vi "SportTrack.vi"() -> ()   [LabVIEW 2023]
uses:
  Global_var.vi
  <vilib>/Utility/NIReport.llb/Report Type.ctl
  <vilib>/Utility/NIReport.llb/NI_ReportGenerationCore.lvlib
  <vilib>/Utility/NIReport.llb/NI_report.lvclass
  <vilib>/addons/_office/NI_ReportGenerationToolkit.lvlib
  <vilib>/addons/_office/word.llb/Word Find & Replace (str).vi
  <vilib>/Utility/NIReport.llb/Word/NI_Word.lvclass
  <vilib>/addons/_office/word.llb/Word Find & Replace (num).vi
  <vilib>/Instr/_visa.llb/VISA Configure Serial Port (Instr).vi
panel:
  out "Buffer vidé\nNe pas lancer tant que ce n'est pas vert constant !":bool
  out "Timer Value":dbl
  out "Execution Time":u32
  in  "stop":bool
  out "String reçu":string
  out "String decouper":string
  in  "OK Button":bool
  in  "time s":dbl min=0.0 max=10.0 step=1.0
  out "?":bool
  in  "acceleration input x (volt)":dbl=1.29 min=0.1 max=2.8 step=0.1
  in  "acceleration input y (volt)":dbl=1.29 min=0.1 max=2.8 step=0.1
  in  "acceleration input z (volt)":dbl=1.35 min=0.1 max=2.8 step=0.1
  out "ACC X":bool
  out "ACC Y":bool
  out "ACC Z":bool
  in  "VISA resource name":refnum<visa-resource-name>="COM7"
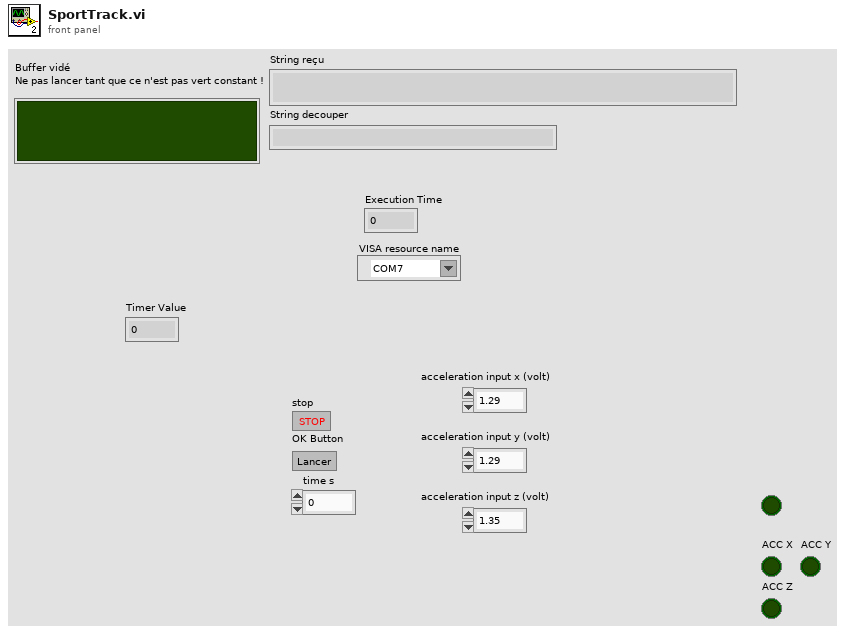
[diagram p1: front panel]
types:
  T1 = enum16{"maximized", "minimized", "normal", "no change"}
  T2 = typedef "NI_ReportGenerationCore.lvlib/Report Type.ctl" = enum16{"HTML", "Word", "Excel"}
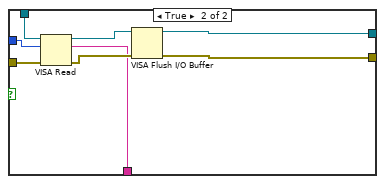
[diagram p2: hidden frame]
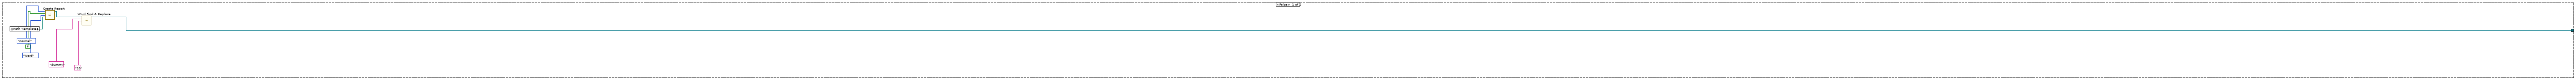
[diagram p4: hidden frame]
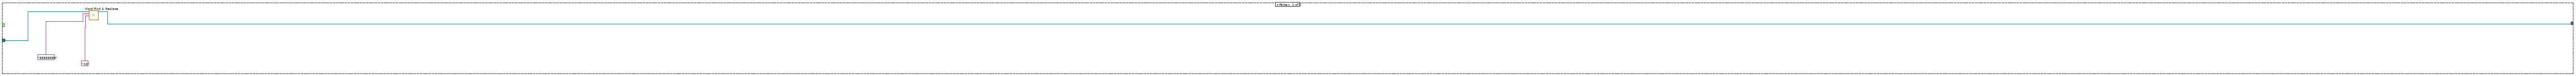
[diagram p5: hidden frame]
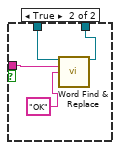
[diagram p6: hidden frame]
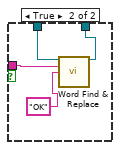
[diagram p7: hidden frame]
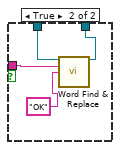
[diagram p8: hidden frame]
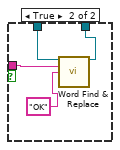
[diagram p9: hidden frame]
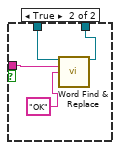
[diagram p10: hidden frame]
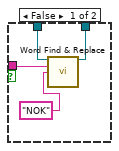
[diagram p11: hidden frame]
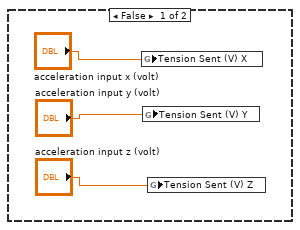
[diagram p12: hidden frame]
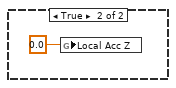
[diagram p13: hidden frame]
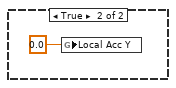
[diagram p14: hidden frame]
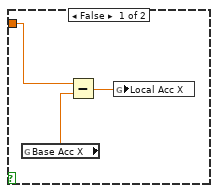
[diagram p15: hidden frame]
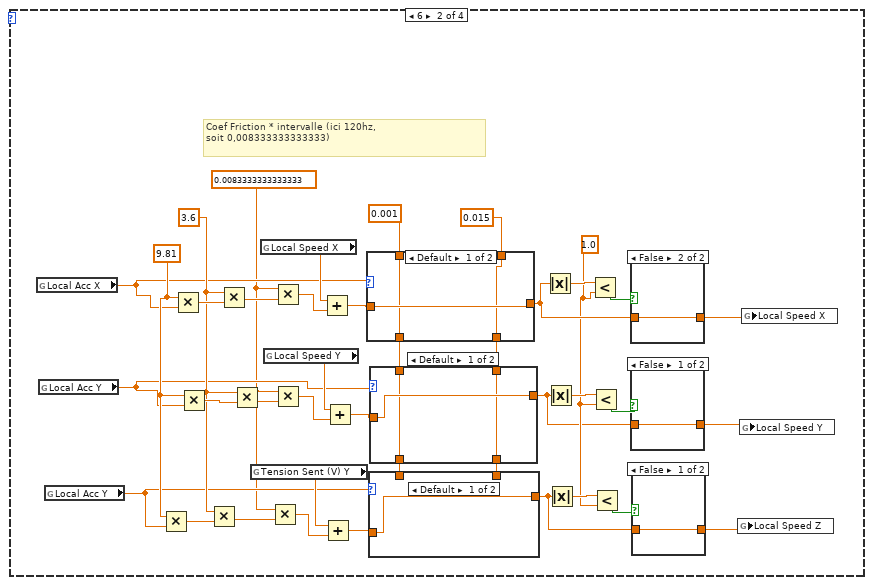
[diagram p17: hidden frame]
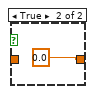
[diagram p18: hidden frame]
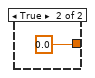
[diagram p19: hidden frame]
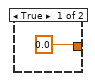
[diagram p20: hidden frame]
diagram:
  w25 = 240.0
  w9 = 0.0
  # "INITIALISATION DES VARIABLES"
  # "0G Voltage Z"
  # "0G Voltage Y"
  # "0G Voltage X"
  n1 = global write "Global_var.vi" "Speed Instant X"(w9) -> ()
  n2 = global write "Global_var.vi" "Speed Instant Y"(w9) -> ()
  n3 = global write "Global_var.vi" "Speed Instant Z"(w9) -> ()
  n4 = global write "Global_var.vi" "Local Speed X"(w9) -> ()
  n5 = global write "Global_var.vi" "Local Speed Y"(w9) -> ()
  n6 = global write "Global_var.vi" "Local Speed Z"(w9) -> ()
  n7 = global write "Global_var.vi" "Local Acc X"(w9) -> ()
  n8 = global write "Global_var.vi" "Local Acc Z"(w9) -> ()
  n9 = global write "Global_var.vi" "Local Acc Y"(w9) -> ()
  n10 = global write "Global_var.vi" "Mesure"(0.0 ("Base Acc Z")) -> ()
  n11 = global write "Global_var.vi" "Acc X"(w9) -> ()
  n12 = global write "Global_var.vi" "Acc Y"(w9) -> ()
  n13 = global write "Global_var.vi" "Acc Z"(w9) -> ()
  n14 = call-poly "VISA Configure Serial Port"("VISA resource name"="VISA resource name", "baud rate (9600)"=115200) -> ("VISA resource name out"=w6:refnum<visa-resource-name>, "error out"=w5:errorcluster)  [unwired: 12 in]
  n15 = global read "Global_var.vi" "Base Tension (V) X"() -> (w10:dbl)
  n16 = global read "Global_var.vi" "Base Tension (V) Z"() -> (w12:dbl)
  n17 = global read "Global_var.vi" "Base Tension (V) Y"() -> (w11:dbl)
  n18 = VISA Clear(VISA resource name=w6, error in (no error)=w5) -> (VISA resource name out=w8:refnum<visa-resource-name>, error out=w7:errorcluster)
  n19 = VISA Open(error in (no error)=w7, VISA resource name=w8) -> (VISA resource name=w3:refnum<visa-resource-name>, error out=w4:errorcluster)  [unwired: 3 in]
  n20 = Current VI's Path() -> (path=w18:path)
  n21 = global write "Global_var.vi" "Base Tension (V) Z"(1.35) -> ()
  n22 = global write "Global_var.vi" "Base Tension (V) Y"(1.29) -> ()
  n23 = global write "Global_var.vi" "Base Tension (V) X"(1.29) -> ()
  n24 = Subtract(x=w11, y=1.29) -> (x-y=w26:dbl)
  n25 = Subtract(x=w10, y=1.29) -> (x-y=w30:dbl)
  n26 = Subtract(x=w12, y=1.35) -> (x-y=w27:dbl)
  n27 = Strip Path(path=w18) -> (stripped path=w21:path)  [unwired: 1 out]
  n28 = Divide(x=w26, y=w25) -> (x/y=w23:dbl)
  n29 = Divide(x=w30, y=w25) -> (x/y=w24:dbl)
  n30 = Divide(x=w27, y=w25) -> (x/y=w22:dbl)
  n31 = VISA Set I/O Buffer Size(VISA resource name=w3, mask (16)=16, size (4096)=5, error in (no error)=w4) -> (VISA resource name out=w2:refnum<visa-resource-name>, error out=w1:errorcluster)
  n32 = global write "Global_var.vi" "Base Acc X"(w24) -> ()
  n33 = global write "Global_var.vi" "Base Acc Y"(w23) -> ()
  n34 = global write "Global_var.vi" "Base Acc Z"(w22) -> ()
  n35 = Build Path(base path=w21, name or relative path=path "Mesures_LabVIEW.docx") -> (appended path=w16:path)
  n36 = Build Path(base path=w21, name or relative path=path "Rapport/Rapport.docx") -> (appended path=w17:path)
  n37 = global write "Global_var.vi" "Path Save"(w17) -> ()
  n38 = global write "Global_var.vi" "Path Template"(w16) -> ()
  n39 = while {
    shift-right: [w46] -> w39
    shift-left: w2 -> [w45]
    shift-right: [w47] -> w38
    shift-left: w1 -> [w44]
    tunnel: [w48] -> w14
    stop <- "stop" stop-if-true
    n40 = flat-sequence {
      tunnel: [w54] -> w51
      tunnel: [w99] -> w48
      tunnel: [w76] -> w46
      tunnel: [w75] -> w47
      tunnel: w43 -> [w60]
      tunnel: w42 -> [w61]
      tunnel: w41 -> [w59]
      tunnel: [w633] -> w52
      frame #0 {
        # "Starting Ticks"
        n41 = Tick Count (ms)() -> (millisecond timer value=w54:u32)
      }
      frame #1 {
        w150 = 0.05
        w162 = 0.05
        w174 = 0.05
        w182 = 0.24
        # "Acc z"
        # "mode"
        # "Acc y"
        # "Acc x"
        # "Speed z"
        # "Speed y"
        # "Speed x"
        # "valeurs en variable"
        # "CALCUL VITESSE"
        # "CALCUL ACCELERATION"
        n42 = Greater?(x=w60, y=100) -> (0:w64:bool)
        n43 = global read "Global_var.vi" "Tension Sent (V) Z"() -> (w86:dbl)
        n44 = global read "Global_var.vi" "Tension Sent (V) Y"() -> (w85:dbl)
        n45 = global read "Global_var.vi" "Tension Sent (V) X"() -> (w84:dbl)
        n46 = local read "String reçu"() -> (w58:string)
        n47 = Subtract(x=w85, y=1.29) -> (x-y=w183:dbl)
        n48 = Subtract(x=w86, y=1.35) -> (x-y=w184:dbl)
        n49 = Subtract(x=w84, y=1.29) -> (x-y=w187:dbl)
        n50 = global read "Global_var.vi" "Base Acc X"() -> (w170:dbl)
        n51 = Divide(x=w187, y=w182) -> (x/y=w83:dbl)
        n52 = Divide(x=w183, y=w182) -> (x/y=w81:dbl)
        n53 = Divide(x=w184, y=w182) -> (x/y=w79:dbl)
        n54 = global read "Global_var.vi" "Base Acc Y"() -> (w158:dbl)
        n55 = global read "Global_var.vi" "Base Acc Z"() -> (w146:dbl)
        n56 = call <vilib>:"Trim Whitespace.vi"("string"=w58) -> ("trimmed string"=w144:string)  [unwired: 1 in]
        n57 = Absolute Value(x=w170) -> (abs(x)=w179:dbl)
        n58 = Absolute Value(x=w170) -> (abs(x)=w181:dbl)
        n59 = Absolute Value(x=w158) -> (abs(x)=w167:dbl)
        n60 = Absolute Value(x=w158) -> (abs(x)=w169:dbl)
        n61 = Match Pattern(string=w144, regular expression="x:") -> (before substring=w67:string, after substring=w141:string)  [unwired: 1 in, 2 out]
        n62 = Equal?(x="SI: ", y=w67) -> (x = y?=w62:bool)
        n63 = And(x=w64, y=w62) -> (x .and. y?=w57:bool)
        n64 = Not(x=w57) -> (.not. x?=→"Buffer vidé\nNe pas lancer tant que ce n'est pas vert constant !":bool)
        n65 = case shown="False" w57 {
          tunnel: [w191 w202] -> w66
          tunnel: [w190 w201] -> w65
          tunnel: w61 -> [w193 w200]
          tunnel: w60 -> [w192 w199]
          tunnel: w59 -> [w194 w198]
          tunnel: [w189 w195] -> w55
          frame False {
            n66 = VISA Read(VISA resource name=w194, byte count=w192, error in (no error)=w193) -> (VISA resource name out=w190:refnum<visa-resource-name>, read buffer=w189:string, error out=w191:errorcluster)  [unwired: 1 out]
          }
          frame True {
            n67 = VISA Read(VISA resource name=w198, byte count=w199, error in (no error)=w200) -> (VISA resource name out=w196:refnum<visa-resource-name>, read buffer=w195:string, error out=w197:errorcluster)  [unwired: 1 out]
            n68 = VISA Flush I/O Buffer(VISA resource name=w196, error in (no error)=w197) -> (VISA resource name out=w201:refnum<visa-resource-name>, error out=w202:errorcluster)  [unwired: 1 in]
          }
        }
        "String reçu" <- w55
        n69 = Multiply(x=1.05, y=w179) -> (x*y=w177:dbl)
        n70 = Multiply(x=0.95, y=w181) -> (x*y=w176:dbl)
        n71 = Absolute Value(x=w146) -> (abs(x)=w155:dbl)
        n72 = Absolute Value(x=w146) -> (abs(x)=w157:dbl)
        n73 = Multiply(x=1.05, y=w167) -> (x*y=w165:dbl)
        n74 = Multiply(x=0.95, y=w169) -> (x*y=w164:dbl)
        n75 = Multiply(x=1.05, y=w155) -> (x*y=w153:dbl)
        n76 = Subtract(x=w174, y=w176) -> (x-y=w175:dbl)
        n77 = Add(x=w174, y=w177) -> (x+y=w171:dbl)
        n78 = Multiply(x=0.95, y=w157) -> (x*y=w152:dbl)
        n79 = Absolute Value(x=w83) -> (abs(x)=w82:dbl)
        n80 = Subtract(x=w162, y=w164) -> (x-y=w163:dbl)
        n81 = Add(x=w162, y=w165) -> (x+y=w159:dbl)
        n82 = Subtract(x=w150, y=w152) -> (x-y=w151:dbl)
        n83 = Add(x=w150, y=w153) -> (x+y=w147:dbl)
        n84 = Absolute Value(x=w81) -> (abs(x)=w80:dbl)
        n85 = call <vilib>:"Trim Whitespace.vi"("string"=w141) -> ("trimmed string"=w140:string)  [unwired: 1 in]
        n86 = Match Pattern(string=w140, regular expression="y:") -> (before substring=w97:string, after substring=w137:string)  [unwired: 1 in, 2 out]
        n87 = call <vilib>:"Trim Whitespace.vi"("string"=w137) -> ("trimmed string"=w138:string)  [unwired: 1 in]
        n88 = Match Pattern(string=w138, regular expression="z:") -> (before substring=w96:string, after substring=w132:string)  [unwired: 1 in, 2 out]
        n89 = call <vilib>:"Trim Whitespace.vi"("string"=w132) -> ("trimmed string"=w135:string)  [unwired: 1 in]
        n90 = Match Pattern(string=w135, regular expression="A: x:") -> (before substring=w95:string, after substring=w131:string)  [unwired: 1 in, 2 out]
        n91 = call <vilib>:"Trim Whitespace.vi"("string"=w131) -> ("trimmed string"=w133:string)  [unwired: 1 in]
        n92 = Match Pattern(string=w133, regular expression="y:") -> (before substring=w98:string, after substring=w129:string)  [unwired: 1 in, 2 out]
        n93 = call <vilib>:"Trim Whitespace.vi"("string"=w129) -> ("trimmed string"=w122:string)  [unwired: 1 in]
        n94 = Match Pattern(string=w122, regular expression="z:") -> (before substring=w69:string, after substring=w121:string)  [unwired: 1 in, 2 out]
        n95 = call <vilib>:"Trim Whitespace.vi"("string"=w121) -> ("trimmed string"=w120:string)  [unwired: 1 in]
        n96 = Match Pattern(string=w120, regular expression="M:") -> (before substring=w70:string, after substring=w119:string)  [unwired: 1 in, 2 out]
        n97 = Absolute Value(x=w79) -> (abs(x)=w78:dbl)
        n98 = Greater Or Equal?(x=w82, y=w175) -> (x >= y?=w172:bool)
        n99 = Less Or Equal?(x=w82, y=w171) -> (x <= y?=w173:bool)
        n100 = Greater Or Equal?(x=w80, y=w163) -> (x >= y?=w160:bool)
        n101 = Less Or Equal?(x=w80, y=w159) -> (x <= y?=w161:bool)
        n102 = And(x=w173, y=w172) -> (x .and. y?=w104:bool)
        "ACC X" <- w104
        n103 = Greater Or Equal?(x=w78, y=w151) -> (x >= y?=w148:bool)
        n104 = Less Or Equal?(x=w78, y=w147) -> (x <= y?=w149:bool)
        n105 = And(x=w161, y=w160) -> (x .and. y?=w105:bool)
        "ACC Y" <- w105
        n106 = And(x=w149, y=w148) -> (x .and. y?=w106:bool)
        "ACC Z" <- w106
        n107 = Concatenate Strings(w97, w96, w95, w98, w69, w70, w119) -> (→"String decouper":string)
        n108 = case shown="True" w104 {
          tunnel: w83 -> [w494 _]
          frame False {
            n109 = global read "Global_var.vi" "Base Acc X"() -> (w493:dbl)
            n110 = Subtract(x=w494, y=w493) -> (x-y=w495:dbl)
            n111 = global write "Global_var.vi" "Local Acc X"(w495) -> ()
          }
          frame True {
            n112 = global write "Global_var.vi" "Local Acc X"(0.0) -> ()
          }
        }
        n113 = case shown="False" w106 {
          tunnel: w79 -> [w486 _]
          frame False {
            n114 = global read "Global_var.vi" "Base Acc Z"() -> (w485:dbl)
            n115 = Subtract(x=w486, y=w485) -> (x-y=w487:dbl)
            n116 = global write "Global_var.vi" "Local Acc Z"(w487) -> ()
          }
          frame True {
            n117 = global write "Global_var.vi" "Local Acc Z"(0.0) -> ()
          }
        }
        n118 = case shown="False" w105 {
          tunnel: w81 -> [w490 _]
          frame False {
            n119 = global read "Global_var.vi" "Base Acc Y"() -> (w489:dbl)
            n120 = Subtract(x=w490, y=w489) -> (x-y=w491:dbl)
            n121 = global write "Global_var.vi" "Local Acc Y"(w491) -> ()
          }
          frame True {
            n122 = global write "Global_var.vi" "Local Acc Y"(0.0) -> ()
          }
        }
        n123 = String Subset(string=w119) -> (substring=w127:string)  [unwired: 2 in]
        n124 = Fract/Exp String To Number(use system decimal point (T)=FALSE, string=w98) -> (number=w113:dbl)  [unwired: 2 in, 1 out]
        n125 = Fract/Exp String To Number(use system decimal point (T)=FALSE, string=w95) -> (number=w112:dbl)  [unwired: 2 in, 1 out]
        n126 = Fract/Exp String To Number(use system decimal point (T)=FALSE, string=w69) -> (number=w114:dbl)  [unwired: 2 in, 1 out]
        n127 = Fract/Exp String To Number(use system decimal point (T)=FALSE, string=w70) -> (number=w115:dbl)  [unwired: 2 in, 1 out]
        n128 = Fract/Exp String To Number(use system decimal point (T)=FALSE, string=w97) -> (number=w71:dbl)  [unwired: 2 in, 1 out]
        n129 = Fract/Exp String To Number(use system decimal point (T)=FALSE, string=w96) -> (number=w111:dbl)  [unwired: 2 in, 1 out]
        n130 = Decimal String To Number(string=w127) -> (number=w116:i32)  [unwired: 2 in, 1 out]
        n131 = global write "Global_var.vi" "Acc Z"(w115) -> ()
        n132 = global write "Global_var.vi" "Acc Y"(w114) -> ()
        n133 = global write "Global_var.vi" "Acc X"(w113) -> ()
        n134 = global write "Global_var.vi" "Mode ACT"(w116) -> ()
        n135 = global write "Global_var.vi" "Speed Instant Y"(w111) -> ()
        n136 = global write "Global_var.vi" "Speed Instant Z"(w112) -> ()
        n137 = global write "Global_var.vi" "Speed Instant X"(w71) -> ()
        n138 = global read "Global_var.vi" "Mode ACT"() -> (w102:dbl)
        n139 = Greater Or Equal?(x=w102, y=4) -> (x >= y?=w101:bool)
        n140 = global read "Global_var.vi" "Mode ACT"() -> (w145:dbl)
        n141 = case shown="4" w145 {
          frame 0, Default {
          }
          frame 6 {
            w497 = 0.0083333333333333
            w515 = 1.0
            w529 = 3.6
            w530 = 9.81
            # "Coef Friction * intervalle (ici 120hz, \nsoit 0,008333333333333)"
            n142 = global read "Global_var.vi" "Local Acc X"() -> (w499:dbl)
            n143 = global read "Global_var.vi" "Local Acc Y"() -> (w500:dbl)
            n144 = global read "Global_var.vi" "Local Acc Y"() -> (w498:dbl)
            n145 = Multiply(x=w530, y=w498) -> (x*y=w531:dbl)
            n146 = Multiply(x=w530, y=w499) -> (x*y=w535:dbl)
            n147 = Multiply(x=w530, y=w500) -> (x*y=w533:dbl)
            n148 = Multiply(x=w529, y=w531) -> (x*y=w532:dbl)
            n149 = Multiply(x=w529, y=w535) -> (x*y=w536:dbl)
            n150 = Multiply(x=w529, y=w533) -> (x*y=w534:dbl)
            n151 = global read "Global_var.vi" "Tension Sent (V) Y"() -> (w505:dbl)
            n152 = global read "Global_var.vi" "Local Speed X"() -> (w512:dbl)
            n153 = global read "Global_var.vi" "Local Speed Y"() -> (w508:dbl)
            n154 = Multiply(x=w497, y=w532) -> (x*y=w506:dbl)
            n155 = Multiply(x=w497, y=w536) -> (x*y=w511:dbl)
            n156 = Multiply(x=w497, y=w534) -> (x*y=w509:dbl)
            n157 = Add(x=w512, y=w511) -> (x+y=w510:dbl)
            n158 = Add(x=w505, y=w506) -> (x+y=w504:dbl)
            n159 = Add(x=w508, y=w509) -> (x+y=w507:dbl)
            n160 = case shown="Default" w499 {
              tunnel: 0.001 -> [w558 w562]
              tunnel: w510 -> [w559 w564]
              tunnel: 0.015 -> [w557 w561]
              tunnel: [w558 w562] -> w526
              tunnel: [w557 w561] -> w524
              tunnel: [w559 w560] -> w522
              frame Default {
              }
              frame 0 {
                n161 = Multiply(x=w562, y=w564) -> (x*y=w563:dbl)
                n162 = Subtract(x=w563, y=w561) -> (x-y=w560:dbl)
              }
            }
            n163 = case shown="Default" w500 {
              tunnel: w526 -> [w549 w555]
              tunnel: [w549 w555] -> w525
              tunnel: w507 -> [w551 w554]
              tunnel: w524 -> [w550 w553]
              tunnel: [w550 w553] -> w523
              tunnel: [w551 w552] -> w513
              frame Default {
              }
              frame 0 {
                n164 = Multiply(x=w555, y=w554) -> (x*y=w556:dbl)
                n165 = Subtract(x=w556, y=w553) -> (x-y=w552:dbl)
              }
            }
            n166 = case shown="Default" w498 {
              tunnel: w525 -> [_ w547]
              tunnel: w504 -> [w543 w546]
              tunnel: w523 -> [_ w545]
              tunnel: [w543 w544] -> w514
              frame Default {
              }
              frame 0 {
                n167 = Multiply(x=w547, y=w546) -> (x*y=w548:dbl)
                n168 = Subtract(x=w548, y=w545) -> (x-y=w544:dbl)
              }
            }
            n169 = Absolute Value(x=w522) -> (abs(x)=w521:dbl)
            n170 = Absolute Value(x=w513) -> (abs(x)=w519:dbl)
            n171 = Absolute Value(x=w514) -> (abs(x)=w517:dbl)
            n172 = Less?(x=w521, y=w515) -> (x < y?=w520:bool)
            n173 = Less?(x=w519, y=w515) -> (x < y?=w518:bool)
            n174 = Less?(x=w517, y=w515) -> (x < y?=w516:bool)
            n175 = case shown="False" w520 {
              tunnel: w522 -> [_ w542]
              tunnel: [0.0 w542] -> w503
              frame True {
              }
              frame False {
              }
            }
            n176 = case shown="False" w518 {
              tunnel: w513 -> [w539 _]
              tunnel: [w539 0.0] -> w502
              frame False {
              }
              frame True {
              }
            }
            n177 = case shown="False" w516 {
              tunnel: w514 -> [w537 _]
              tunnel: [w537 0.0] -> w501
              frame False {
              }
              frame True {
              }
            }
            n178 = global write "Global_var.vi" "Local Speed Z"(w501) -> ()
            n179 = global write "Global_var.vi" "Local Speed Y"(w502) -> ()
            n180 = global write "Global_var.vi" "Local Speed X"(w503) -> ()
          }
          frame 2 {
          }
          frame 4 {
            w582 = 1.0
            w597 = 3.6
            w598 = 9.81
            w596 = 0.1
            # "Coef Friction * intervalle (ici 10hz, soit 0.1)"
            n181 = global read "Global_var.vi" "Local Acc X"() -> (w567:dbl)
            n182 = global read "Global_var.vi" "Local Acc Y"() -> (w566:dbl)
            n183 = global read "Global_var.vi" "Local Acc Y"() -> (w565:dbl)
            n184 = Multiply(x=w598, y=w565) -> (x*y=w599:dbl)
            n185 = Multiply(x=w598, y=w567) -> (x*y=w603:dbl)
            n186 = Multiply(x=w598, y=w566) -> (x*y=w601:dbl)
            n187 = Multiply(x=w597, y=w599) -> (x*y=w600:dbl)
            n188 = Multiply(x=w597, y=w603) -> (x*y=w604:dbl)
            n189 = Multiply(x=w597, y=w601) -> (x*y=w602:dbl)
            n190 = global read "Global_var.vi" "Local Speed X"() -> (w579:dbl)
            n191 = global read "Global_var.vi" "Local Speed Z"() -> (w572:dbl)
            n192 = global read "Global_var.vi" "Local Speed Y"() -> (w575:dbl)
            n193 = Multiply(x=w596, y=w600) -> (x*y=w573:dbl)
            n194 = Multiply(x=w596, y=w604) -> (x*y=w578:dbl)
            n195 = Multiply(x=w596, y=w602) -> (x*y=w576:dbl)
            n196 = Add(x=w579, y=w578) -> (x+y=w577:dbl)
            n197 = Add(x=w572, y=w573) -> (x+y=w571:dbl)
            n198 = Add(x=w575, y=w576) -> (x+y=w574:dbl)
            n199 = case shown="0" w567 {
              tunnel: 0.001 -> [w626 w630]
              tunnel: w577 -> [w627 w632]
              tunnel: 0.015 -> [w625 w629]
              tunnel: [w626 w630] -> w593
              tunnel: [w625 w629] -> w591
              tunnel: [w627 w628] -> w589
              frame Default {
              }
              frame 0 {
                n200 = Multiply(x=w630, y=w632) -> (x*y=w631:dbl)
                n201 = Subtract(x=w631, y=w629) -> (x-y=w628:dbl)
              }
            }
            n202 = case shown="0" w566 {
              tunnel: w593 -> [w617 w623]
              tunnel: [w617 w623] -> w592
              tunnel: w574 -> [w619 w622]
              tunnel: w591 -> [w618 w621]
              tunnel: [w618 w621] -> w590
              tunnel: [w619 w620] -> w580
              frame Default {
              }
              frame 0 {
                n203 = Multiply(x=w623, y=w622) -> (x*y=w624:dbl)
                n204 = Subtract(x=w624, y=w621) -> (x-y=w620:dbl)
              }
            }
            n205 = case shown="0" w565 {
              tunnel: w592 -> [_ w615]
              tunnel: w571 -> [w611 w614]
              tunnel: w590 -> [_ w613]
              tunnel: [w611 w612] -> w581
              frame Default {
              }
              frame 0 {
                n206 = Multiply(x=w615, y=w614) -> (x*y=w616:dbl)
                n207 = Subtract(x=w616, y=w613) -> (x-y=w612:dbl)
              }
            }
            n208 = Absolute Value(x=w589) -> (abs(x)=w588:dbl)
            n209 = Absolute Value(x=w580) -> (abs(x)=w586:dbl)
            n210 = Absolute Value(x=w581) -> (abs(x)=w584:dbl)
            n211 = Less?(x=w588, y=w582) -> (x < y?=w587:bool)
            n212 = Less?(x=w586, y=w582) -> (x < y?=w585:bool)
            n213 = Less?(x=w584, y=w582) -> (x < y?=w583:bool)
            n214 = case shown="True" w587 {
              tunnel: w589 -> [_ w610]
              tunnel: [0.0 w610] -> w570
              frame True {
              }
              frame False {
              }
            }
            n215 = case shown="True" w585 {
              tunnel: w580 -> [w607 _]
              tunnel: [w607 0.0] -> w569
              frame False {
              }
              frame True {
              }
            }
            n216 = case shown="True" w583 {
              tunnel: w581 -> [w605 _]
              tunnel: [w605 0.0] -> w568
              frame False {
              }
              frame True {
              }
            }
            n217 = global write "Global_var.vi" "Local Speed Z"(w568) -> ()
            n218 = global write "Global_var.vi" "Local Speed Y"(w569) -> ()
            n219 = global write "Global_var.vi" "Local Speed X"(w570) -> ()
          }
        }
        n220 = And(x="OK Button", y=w101) -> (x .and. y?=w77:bool)
        n221 = case shown="True" w77 {
          tunnel: w65 -> [w204 w208]
          tunnel: [w204 w207] -> w76
          tunnel: w66 -> [w203 w206]
          tunnel: [w203 w205] -> w75
          frame False {
          }
          frame True {
            n222 = VISA Flush I/O Buffer(VISA resource name=w208, error in (no error)=w206) -> (VISA resource name out=w207:refnum<visa-resource-name>, error out=w205:errorcluster)  [unwired: 1 in]
          }
        }
        n223 = Multiply(x="time s", y=2.0) -> (x*y=w88:dbl)
        n224 = call "Elapsed Time"("Time Target (s)"="time s", "Reset"=w77, "Auto Reset"=FALSE) -> ("Elapsed Time (s)"=w72:dbl, "Time has Elapsed"=w125:bool)  [unwired: 9 in, 6 out]
        "Timer Value" <- w72
        n225 = Less Or Equal?(x=w72, y=w88) -> (x <= y?=w87:bool)
        "?" <- w87
        n226 = case shown="True" w87 {
          tunnel: w77 -> [_ w230]
          tunnel: [w209 w217] -> w99
          tunnel: w88 -> [_ w220]
          tunnel: w87 -> [_ w218]
          frame False {
            n227 = global read "Global_var.vi" "Path Template"() -> (w216:path)
            n228 = call <vilib>:"Create Report.vi"("window state (normal)"=T1."normal", "display alerts? (F)"=FALSE, "report type"=Report_Type."Word", "template (empty)"=w216) -> ("report out"=w211:refnum<class "NI_report.lvclass">)  [unwired: 10 in, 1 out]
            n229 = call-poly <vilib>:"Word Find & Replace.vi"("report in"=w211, "find what?"="dummy", "replace with"="10") -> ("report out"=w209:refnum<class "NI_report.lvclass">)  [unwired: 10 in, 2 out]
          }
          frame True {
            n230 = Divide(x=w220, y=20.0) -> (x/y=w219:dbl)
            n231 = global read "Global_var.vi" "Path Template"() -> (w228:path)
            n232 = call "Elapsed Time2"("Time Target (s)"=w219, "Reset"=w230, "Auto Reset"=TRUE) -> ("Time has Elapsed"=w222:bool)  [unwired: 9 in, 7 out]
            n233 = And(x=w218, y=w222) -> (x .and. y?=w223:bool)
            n234 = call <vilib>:"Create Report.vi"("window state (normal)"=T1."normal", "display alerts? (F)"=FALSE, "report type"=Report_Type."Word", "template (empty)"=w228) -> ("report out"=w229:refnum<class "NI_report.lvclass">)  [unwired: 10 in, 1 out]
            n235 = case shown="True" w223 {
              tunnel: w229 -> [w234 w430]
              tunnel: [w231 w266] -> w217
              frame False {
                n236 = call-poly <vilib>:"Word Find & Replace.vi"("report in"=w234, "find what?"="85858585", "replace with"="10") -> ("report out"=w231:refnum<class "NI_report.lvclass">)  [unwired: 10 in, 2 out]
              }
              frame True {
                n237 = global read "Global_var.vi" "Mesure"() -> (w425:dbl)
                n238 = Number To Decimal String(number=w425) -> (decimal integer string=w426:string)  [unwired: 1 in]
                n239 = global read "Global_var.vi" "Mesure"() -> (w428:dbl)
                n240 = Concatenate Strings("MAX" ("find what?"), w426) -> (w424:string)
                n241 = Add(x=w428, y=1) -> (x+y=w356:dbl)
                n242 = global read "Global_var.vi" "Acc X"() -> (w423:dbl)
                n243 = call-poly <vilib>:"Word Find & Replace.vi"("report in"=w430, "find what?"=w424, "replace with"=w423) -> ("report out"=w397:refnum<class "NI_report.lvclass">)  [unwired: 10 in, 2 out]
                n244 = global read "Global_var.vi" "Mesure"() -> (w420:dbl)
                n245 = global write "Global_var.vi" "Mesure"(w356) -> ()
                n246 = Number To Decimal String(number=w420) -> (decimal integer string=w421:string)  [unwired: 1 in]
                n247 = Concatenate Strings("VRAX" ("find what?"), w421) -> (w418:string)
                n248 = global read "Global_var.vi" "Local Acc X"() -> (w419:dbl)
                n249 = call-poly <vilib>:"Word Find & Replace.vi"("report in"=w397, "find what?"=w418, "replace with"=w419) -> ("report out"=w400:refnum<class "NI_report.lvclass">)  [unwired: 10 in, 2 out]
                n250 = global read "Global_var.vi" "Mesure"() -> (w415:dbl)
                n251 = Number To Decimal String(number=w415) -> (decimal integer string=w416:string)  [unwired: 1 in]
                n252 = Concatenate Strings("MAY" ("find what?"), w416) -> (w401:string)
                n253 = global read "Global_var.vi" "Acc Y"() -> (w414:dbl)
                n254 = call-poly <vilib>:"Word Find & Replace.vi"("report in"=w400, "find what?"=w401, "replace with"=w414) -> ("report out"=w398:refnum<class "NI_report.lvclass">)  [unwired: 10 in, 2 out]
                n255 = global read "Global_var.vi" "Mesure"() -> (w411:dbl)
                n256 = Number To Decimal String(number=w411) -> (decimal integer string=w412:string)  [unwired: 1 in]
                n257 = Concatenate Strings("VRAY" ("find what?"), w412) -> (w399:string)
                n258 = global read "Global_var.vi" "Local Acc Y"() -> (w410:dbl)
                n259 = call-poly <vilib>:"Word Find & Replace.vi"("report in"=w398, "find what?"=w399, "replace with"=w410) -> ("report out"=w395:refnum<class "NI_report.lvclass">)  [unwired: 10 in, 2 out]
                n260 = global read "Global_var.vi" "Mesure"() -> (w407:dbl)
                n261 = Number To Decimal String(number=w407) -> (decimal integer string=w408:string)  [unwired: 1 in]
                n262 = Concatenate Strings("MAZ" ("find what?"), w408) -> (w396:string)
                n263 = global read "Global_var.vi" "Acc Z"() -> (w406:dbl)
                n264 = call-poly <vilib>:"Word Find & Replace.vi"("report in"=w395, "find what?"=w396, "replace with"=w406) -> ("report out"=w393:refnum<class "NI_report.lvclass">)  [unwired: 10 in, 2 out]
                n265 = global read "Global_var.vi" "Mesure"() -> (w403:dbl)
                n266 = Number To Decimal String(number=w403) -> (decimal integer string=w404:string)  [unwired: 1 in]
                n267 = Concatenate Strings("VRAZ" ("find what?"), w404) -> (w394:string)
                n268 = global read "Global_var.vi" "Local Acc Z"() -> (w402:dbl)
                n269 = call-poly <vilib>:"Word Find & Replace.vi"("report in"=w393, "find what?"=w394, "replace with"=w402) -> ("report out"=w357:refnum<class "NI_report.lvclass">)  [unwired: 10 in, 2 out]
                n270 = global read "Global_var.vi" "Mesure"() -> (w390:dbl)
                n271 = Number To Decimal String(number=w390) -> (decimal integer string=w391:string)  [unwired: 1 in]
                n272 = Concatenate Strings("MVX" ("find what?"), w391) -> (w389:string)
                n273 = global read "Global_var.vi" "Speed Instant X"() -> (w388:dbl)
                n274 = call-poly <vilib>:"Word Find & Replace.vi"("report in"=w357, "find what?"=w389, "replace with"=w388) -> ("report out"=w362:refnum<class "NI_report.lvclass">)  [unwired: 10 in, 2 out]
                n275 = global read "Global_var.vi" "Mesure"() -> (w385:dbl)
                n276 = Number To Decimal String(number=w385) -> (decimal integer string=w386:string)  [unwired: 1 in]
                n277 = Concatenate Strings("VRVX" ("find what?"), w386) -> (w383:string)
                n278 = global read "Global_var.vi" "Local Speed X"() -> (w384:dbl)
                n279 = call-poly <vilib>:"Word Find & Replace.vi"("report in"=w362, "find what?"=w383, "replace with"=w384) -> ("report out"=w365:refnum<class "NI_report.lvclass">)  [unwired: 10 in, 2 out]
                n280 = global read "Global_var.vi" "Mesure"() -> (w380:dbl)
                n281 = Number To Decimal String(number=w380) -> (decimal integer string=w381:string)  [unwired: 1 in]
                n282 = Concatenate Strings("MVY" ("find what?"), w381) -> (w366:string)
                n283 = global read "Global_var.vi" "Speed Instant Y"() -> (w379:dbl)
                n284 = call-poly <vilib>:"Word Find & Replace.vi"("report in"=w365, "find what?"=w366, "replace with"=w379) -> ("report out"=w363:refnum<class "NI_report.lvclass">)  [unwired: 10 in, 2 out]
                n285 = global read "Global_var.vi" "Mesure"() -> (w376:dbl)
                n286 = Number To Decimal String(number=w376) -> (decimal integer string=w377:string)  [unwired: 1 in]
                n287 = Concatenate Strings("VRVY" ("find what?"), w377) -> (w364:string)
                n288 = global read "Global_var.vi" "Local Speed Y"() -> (w375:dbl)
                n289 = call-poly <vilib>:"Word Find & Replace.vi"("report in"=w363, "find what?"=w364, "replace with"=w375) -> ("report out"=w360:refnum<class "NI_report.lvclass">)  [unwired: 10 in, 2 out]
                n290 = global read "Global_var.vi" "Mesure"() -> (w372:dbl)
                n291 = Number To Decimal String(number=w372) -> (decimal integer string=w373:string)  [unwired: 1 in]
                n292 = Concatenate Strings("MVZ" ("find what?"), w373) -> (w361:string)
                n293 = global read "Global_var.vi" "Speed Instant Z"() -> (w371:dbl)
                n294 = call-poly <vilib>:"Word Find & Replace.vi"("report in"=w360, "find what?"=w361, "replace with"=w371) -> ("report out"=w358:refnum<class "NI_report.lvclass">)  [unwired: 10 in, 2 out]
                n295 = global read "Global_var.vi" "Mesure"() -> (w368:dbl)
                n296 = Number To Decimal String(number=w368) -> (decimal integer string=w369:string)  [unwired: 1 in]
                n297 = Concatenate Strings("VRVZ" ("find what?"), w369) -> (w359:string)
                n298 = global read "Global_var.vi" "Local Speed Z"() -> (w367:dbl)
                n299 = call-poly <vilib>:"Word Find & Replace.vi"("report in"=w358, "find what?"=w359, "replace with"=w367) -> ("report out"=w285:refnum<class "NI_report.lvclass">)  [unwired: 10 in, 2 out]
                n300 = global read "Global_var.vi" "Mesure"() -> (w353:dbl)
                n301 = Number To Decimal String(number=w353) -> (decimal integer string=w354:string)  [unwired: 1 in]
                n302 = global read "Global_var.vi" "Local Acc X"() -> (w350:dbl)
                n303 = Concatenate Strings("DAX" ("find what?"), w354) -> (w352:string)
                n304 = global read "Global_var.vi" "Acc X"() -> (w351:dbl)
                n305 = Subtract(x=w351, y=w350) -> (x-y=w264:dbl)
                n306 = Equal?(x=0, y=w264) -> (x = y?=w261:bool)
                n307 = Divide(x=w264, y=w350) -> (x/y=w318:dbl)
                n308 = call-poly <vilib>:"Word Find & Replace.vi"("report in"=w285, "find what?"=w352, "replace with"=w318) -> ("report out"=w311:refnum<class "NI_report.lvclass">)  [unwired: 10 in, 2 out]
                n309 = Absolute Value(x=w318) -> (abs(x)=w317:dbl)
                n310 = global read "Global_var.vi" "Mesure"() -> (w316:dbl)
                n311 = Number To Decimal String(number=w316) -> (decimal integer string=w314:string)  [unwired: 1 in]
                n312 = Less?(x=w317, y=0.05) -> (x < y?=w262:bool)
                n313 = Concatenate Strings("CAX" ("find what?"), w314) -> (w313:string)
                n314 = Or(x=w261, y=w262) -> (x .or. y?=w260:bool)
                n315 = case shown="True" w260 {
                  tunnel: w313 -> [w474 w478]
                  tunnel: [w472 w476] -> w312
                  tunnel: w311 -> [w471 w475]
                  frame False {
                    n316 = call-poly <vilib>:"Word Find & Replace.vi"("report in"=w471, "find what?"=w474, "replace with"="NOK") -> ("report out"=w472:refnum<class "NI_report.lvclass">)  [unwired: 10 in, 2 out]
                  }
                  frame True {
                    n317 = call-poly <vilib>:"Word Find & Replace.vi"("report in"=w475, "find what?"=w478, "replace with"="OK") -> ("report out"=w476:refnum<class "NI_report.lvclass">)  [unwired: 10 in, 2 out]
                  }
                }
                n318 = global read "Global_var.vi" "Mesure"() -> (w347:dbl)
                n319 = Number To Decimal String(number=w347) -> (decimal integer string=w348:string)  [unwired: 1 in]
                n320 = global read "Global_var.vi" "Local Acc Y"() -> (w344:dbl)
                n321 = Concatenate Strings("DAY" ("find what?"), w348) -> (w346:string)
                n322 = global read "Global_var.vi" "Acc Y"() -> (w345:dbl)
                n323 = Subtract(x=w345, y=w344) -> (x-y=w258:dbl)
                n324 = Equal?(x=0, y=w258) -> (x = y?=w257:bool)
                n325 = Divide(x=w258, y=w344) -> (x/y=w302:dbl)
                n326 = call-poly <vilib>:"Word Find & Replace.vi"("report in"=w312, "find what?"=w346, "replace with"=w302) -> ("report out"=w304:refnum<class "NI_report.lvclass">)  [unwired: 10 in, 2 out]
                n327 = global read "Global_var.vi" "Mesure"() -> (w308:dbl)
                n328 = Absolute Value(x=w302) -> (abs(x)=w309:dbl)
                n329 = Number To Decimal String(number=w308) -> (decimal integer string=w306:string)  [unwired: 1 in]
                n330 = Less?(x=w309, y=0.05) -> (x < y?=w255:bool)
                n331 = Concatenate Strings("CAY" ("find what?"), w306) -> (w305:string)
                n332 = Or(x=w257, y=w255) -> (x .or. y?=w256:bool)
                n333 = case shown="False" w256 {
                  tunnel: w305 -> [w466 w470]
                  tunnel: [w464 w468] -> w303
                  tunnel: w304 -> [w463 w467]
                  frame False {
                    n334 = call-poly <vilib>:"Word Find & Replace.vi"("report in"=w463, "find what?"=w466, "replace with"="NOK") -> ("report out"=w464:refnum<class "NI_report.lvclass">)  [unwired: 10 in, 2 out]
                  }
                  frame True {
                    n335 = call-poly <vilib>:"Word Find & Replace.vi"("report in"=w467, "find what?"=w470, "replace with"="OK") -> ("report out"=w468:refnum<class "NI_report.lvclass">)  [unwired: 10 in, 2 out]
                  }
                }
                n336 = global read "Global_var.vi" "Mesure"() -> (w341:dbl)
                n337 = Number To Decimal String(number=w341) -> (decimal integer string=w342:string)  [unwired: 1 in]
                n338 = global read "Global_var.vi" "Local Acc Z"() -> (w338:dbl)
                n339 = Concatenate Strings("DAZ" ("find what?"), w342) -> (w340:string)
                n340 = global read "Global_var.vi" "Acc Z"() -> (w339:dbl)
                n341 = Subtract(x=w339, y=w338) -> (x-y=w253:dbl)
                n342 = Equal?(x=0, y=w253) -> (x = y?=w252:bool)
                n343 = Divide(x=w253, y=w338) -> (x/y=w293:dbl)
                n344 = call-poly <vilib>:"Word Find & Replace.vi"("report in"=w303, "find what?"=w340, "replace with"=w293) -> ("report out"=w295:refnum<class "NI_report.lvclass">)  [unwired: 10 in, 2 out]
                n345 = global read "Global_var.vi" "Mesure"() -> (w299:dbl)
                n346 = Absolute Value(x=w293) -> (abs(x)=w300:dbl)
                n347 = Number To Decimal String(number=w299) -> (decimal integer string=w297:string)  [unwired: 1 in]
                n348 = Less?(x=w300, y=0.05) -> (x < y?=w251:bool)
                n349 = Concatenate Strings("CAZ" ("find what?"), w297) -> (w296:string)
                n350 = Or(x=w252, y=w251) -> (x .or. y?=w250:bool)
                n351 = case shown="False" w250 {
                  tunnel: w296 -> [w458 w462]
                  tunnel: [w456 w460] -> w294
                  tunnel: w295 -> [w455 w459]
                  frame False {
                    n352 = call-poly <vilib>:"Word Find & Replace.vi"("report in"=w455, "find what?"=w458, "replace with"="NOK") -> ("report out"=w456:refnum<class "NI_report.lvclass">)  [unwired: 10 in, 2 out]
                  }
                  frame True {
                    n353 = call-poly <vilib>:"Word Find & Replace.vi"("report in"=w459, "find what?"=w462, "replace with"="OK") -> ("report out"=w460:refnum<class "NI_report.lvclass">)  [unwired: 10 in, 2 out]
                  }
                }
                n354 = global read "Global_var.vi" "Mesure"() -> (w335:dbl)
                n355 = Number To Decimal String(number=w335) -> (decimal integer string=w336:string)  [unwired: 1 in]
                n356 = global read "Global_var.vi" "Local Speed X"() -> (w332:dbl)
                n357 = Concatenate Strings("DVX" ("find what?"), w336) -> (w334:string)
                n358 = global read "Global_var.vi" "Speed Instant X"() -> (w333:dbl)
                n359 = Subtract(x=w333, y=w332) -> (x-y=w248:dbl)
                n360 = Equal?(x=0, y=w248) -> (x = y?=w247:bool)
                n361 = Divide(x=w248, y=w332) -> (x/y=w283:dbl)
                n362 = call-poly <vilib>:"Word Find & Replace.vi"("report in"=w294, "find what?"=w334, "replace with"=w283) -> ("report out"=w286:refnum<class "NI_report.lvclass">)  [unwired: 10 in, 2 out]
                n363 = Absolute Value(x=w283) -> (abs(x)=w291:dbl)
                n364 = global read "Global_var.vi" "Mesure"() -> (w290:dbl)
                n365 = Number To Decimal String(number=w290) -> (decimal integer string=w288:string)  [unwired: 1 in]
                n366 = Less?(x=w291, y=0.05) -> (x < y?=w246:bool)
                n367 = Concatenate Strings("CVX" ("find what?"), w288) -> (w287:string)
                n368 = Or(x=w247, y=w246) -> (x .or. y?=w245:bool)
                n369 = case shown="False" w245 {
                  tunnel: w287 -> [w450 w454]
                  tunnel: [w448 w452] -> w284
                  tunnel: w286 -> [w447 w451]
                  frame False {
                    n370 = call-poly <vilib>:"Word Find & Replace.vi"("report in"=w447, "find what?"=w450, "replace with"="NOK") -> ("report out"=w448:refnum<class "NI_report.lvclass">)  [unwired: 10 in, 2 out]
                  }
                  frame True {
                    n371 = call-poly <vilib>:"Word Find & Replace.vi"("report in"=w451, "find what?"=w454, "replace with"="OK") -> ("report out"=w452:refnum<class "NI_report.lvclass">)  [unwired: 10 in, 2 out]
                  }
                }
                n372 = global read "Global_var.vi" "Mesure"() -> (w329:dbl)
                n373 = Number To Decimal String(number=w329) -> (decimal integer string=w330:string)  [unwired: 1 in]
                n374 = global read "Global_var.vi" "Local Speed Y"() -> (w326:dbl)
                n375 = Concatenate Strings("DVY" ("find what?"), w330) -> (w328:string)
                n376 = global read "Global_var.vi" "Speed Instant Y"() -> (w327:dbl)
                n377 = Subtract(x=w327, y=w326) -> (x-y=w243:dbl)
                n378 = Equal?(x=0, y=w243) -> (x = y?=w240:bool)
                n379 = Divide(x=w243, y=w326) -> (x/y=w275:dbl)
                n380 = call-poly <vilib>:"Word Find & Replace.vi"("report in"=w284, "find what?"=w328, "replace with"=w275) -> ("report out"=w276:refnum<class "NI_report.lvclass">)  [unwired: 10 in, 2 out]
                n381 = global read "Global_var.vi" "Mesure"() -> (w280:dbl)
                n382 = Absolute Value(x=w275) -> (abs(x)=w281:dbl)
                n383 = Number To Decimal String(number=w280) -> (decimal integer string=w278:string)  [unwired: 1 in]
                n384 = Less?(x=w281, y=0.05) -> (x < y?=w241:bool)
                n385 = Concatenate Strings("CVY" ("find what?"), w278) -> (w277:string)
                n386 = Or(x=w240, y=w241) -> (x .or. y?=w242:bool)
                n387 = case shown="False" w242 {
                  tunnel: w277 -> [w442 w446]
                  tunnel: [w440 w444] -> w274
                  tunnel: w276 -> [w439 w443]
                  frame False {
                    n388 = call-poly <vilib>:"Word Find & Replace.vi"("report in"=w439, "find what?"=w442, "replace with"="NOK") -> ("report out"=w440:refnum<class "NI_report.lvclass">)  [unwired: 10 in, 2 out]
                  }
                  frame True {
                    n389 = call-poly <vilib>:"Word Find & Replace.vi"("report in"=w443, "find what?"=w446, "replace with"="OK") -> ("report out"=w444:refnum<class "NI_report.lvclass">)  [unwired: 10 in, 2 out]
                  }
                }
                n390 = global read "Global_var.vi" "Mesure"() -> (w323:dbl)
                n391 = Number To Decimal String(number=w323) -> (decimal integer string=w324:string)  [unwired: 1 in]
                n392 = global read "Global_var.vi" "Local Speed Z"() -> (w320:dbl)
                n393 = Concatenate Strings("DVZ" ("find what?"), w324) -> (w322:string)
                n394 = global read "Global_var.vi" "Speed Instant Z"() -> (w321:dbl)
                n395 = Subtract(x=w321, y=w320) -> (x-y=w238:dbl)
                n396 = Equal?(x=0, y=w238) -> (x = y?=w237:bool)
                n397 = Divide(x=w238, y=w320) -> (x/y=w265:dbl)
                n398 = call-poly <vilib>:"Word Find & Replace.vi"("report in"=w274, "find what?"=w322, "replace with"=w265) -> ("report out"=w267:refnum<class "NI_report.lvclass">)  [unwired: 10 in, 2 out]
                n399 = global read "Global_var.vi" "Mesure"() -> (w271:dbl)
                n400 = Absolute Value(x=w265) -> (abs(x)=w272:dbl)
                n401 = Number To Decimal String(number=w271) -> (decimal integer string=w269:string)  [unwired: 1 in]
                n402 = Less?(x=w272, y=0.05) -> (x < y?=w235:bool)
                n403 = Concatenate Strings("CVZ" ("find what?"), w269) -> (w268:string)
                n404 = Or(x=w237, y=w235) -> (x .or. y?=w236:bool)
                n405 = case shown="False" w236 {
                  tunnel: w268 -> [w434 w438]
                  tunnel: [w432 w436] -> w266
                  tunnel: w267 -> [w431 w435]
                  frame False {
                    n406 = call-poly <vilib>:"Word Find & Replace.vi"("report in"=w431, "find what?"=w434, "replace with"="NOK") -> ("report out"=w432:refnum<class "NI_report.lvclass">)  [unwired: 10 in, 2 out]
                  }
                  frame True {
                    n407 = call-poly <vilib>:"Word Find & Replace.vi"("report in"=w435, "find what?"=w438, "replace with"="OK") -> ("report out"=w436:refnum<class "NI_report.lvclass">)  [unwired: 10 in, 2 out]
                  }
                }
              }
            }
          }
        }
        n408 = global read "Global_var.vi" "Mode ACT"() -> (w110:dbl)
        n409 = Less Or Equal?(x=w110, y=2) -> (x <= y?=w118:bool)
        n410 = Or(x=w125, y=w118) -> (x .or. y?=w126:bool)
        n411 = case shown="True" w126 {
          frame False {
            n412 = global write "Global_var.vi" "Tension Sent (V) X"("acceleration input x (volt)") -> ()
            n413 = global write "Global_var.vi" "Tension Sent (V) Y"("acceleration input y (volt)") -> ()
            n414 = global write "Global_var.vi" "Tension Sent (V) Z"("acceleration input z (volt)") -> ()
          }
          frame True {
            n415 = global read "Global_var.vi" "Base Tension (V) Y"() -> (w483:dbl)
            n416 = global read "Global_var.vi" "Base Tension (V) X"() -> (w482:dbl)
            n417 = global read "Global_var.vi" "Base Tension (V) Z"() -> (w484:dbl)
            n418 = global write "Global_var.vi" "Tension Sent (V) X"(w482) -> ()
            n419 = global write "Global_var.vi" "Tension Sent (V) Y"(w483) -> ()
            n420 = global write "Global_var.vi" "Tension Sent (V) Z"(w484) -> ()
          }
        }
        n421 = global read "Global_var.vi" "Tension Sent (V) X"() -> (w109:dbl)
        n422 = global read "Global_var.vi" "Tension Sent (V) Y"() -> (w107:dbl)
        n423 = global read "Global_var.vi" "Tension Sent (V) Z"() -> (w108:dbl)
        n424 = shared-variable "cRIO-9063\\Mod1\\AO0"(w109) -> ()  [unwired: 1 in, 1 out]
        n425 = shared-variable "cRIO-9063\\Mod1\\AO2"(w108) -> ()  [unwired: 1 in, 1 out]
        n426 = shared-variable "cRIO-9063\\Mod1\\AO1"(w107) -> ()  [unwired: 1 in, 1 out]
      }
      frame #2 {
        # "Ending Ticks"
        n427 = Tick Count (ms)() -> (millisecond timer value=w633:u32)
      }
    }
    n428 = property class="Instr"(reference=w45, error in=w44) -> (reference out=w41:refnum<visa-resource-name>, error out=w42:errorcluster, "Bytes at Port"=w43:u32)
    n429 = Wait (ms)(milliseconds to wait=u32 75) -> ()  [unwired: 1 out]
    n430 = Subtract(x=w52, y=w51) -> (x-y=→"Execution Time":u32)
  }
  n431 = global read "Global_var.vi" "Path Save"() -> (w15:path)
  n432 = call-dynamic "Save Report to File.vi"("report in"=w14, "report file path"=w15) -> ()  [unwired: 12 in, 2 out]
  n433 = VISA Close(VISA resource name=w39, error in (no error)=w38) -> ()  [unwired: 1 out]
